vi "S4CCS.vi"() -> ()   [LabVIEW 2018]
uses:
  Channel/Channel.lvclass
  Channel/Channel.lvclass/Channel.ctl
  Header content/Header content.lvclass/Header content.ctl
  Server/Server.lvclass/Server.ctl
  Simulated_CCD_Camera/Simulated Camera.lvclass/Simulated Camera.ctl
  State Machine/CCS_State Machine.lvclass
  RxTx/CCS_RxTx.lvclass
  Simulated_CCD_Camera/Simulated Camera.lvclass
  Header content/Header content.lvclass
  Log File/CCS_Log File.lvclass
  Error log/Error log.lvclass
  Keywords Log File/Keywords Log File.lvclass
  Server/Server.lvclass
  <userlib>/gfitsio/gfitsio-read-image-subset-i32-2d.vi
panel:
  out "error out":errorcluster
  in  "Tab Control":T1(tab)
  out "S4GUI":bool
  out "S4ICS":bool
  out "TCS":bool
  out "Weather Station":bool
  out "Focuser":bool
  in  "Configuration to initialize ACS":T2={"Image path"=path "C:/images/today", "Remote IP"="200.131.64.25", "Channel"=1, "ACS mode"=0, "Communication"=0} {"Communication" items=["ZeroMQ", "TCP-IP"]; "ACS mode" items=["simulated", "real"]; "Channel" min=1 max=4}
  out "Wait expose cmd":bool
  in  "Stop Button":bool
  in  "Software version":string="v1.51.2"
  out "CCD ON/OFF":bool
  in  "use config file":bool=TRUE
  out "Acquiring 3":bool
  out "Numeric 2":i32
  out "Error Message":string
  out "Acquiring 2":bool
  out "Numeric":i32
  out "Code error message":string
  in  "clean error":bool
  out "#cycles":u32
  out "cycles done":u16
  out "#seqs":u32
  out "seqs done":u16
  out "last update":string
  out "S4GUI Message":string
  out "Last image":string
  out "frames done":u16
  out "CCD status":string
  out "Temperature (ºC)":i16
  out "Temperature status":string
  out "exptime (s)":dbl
  out "Serial number":u16
  out "Acquiring":bool
  out "#frames":u32
  in  "video mode":bool
  in  "reset axis":bool
  in  "contrast":dbl(slide)=1.0 scale=0.0..1.0
  in  "counts level":dbl(slide)=15.0 scale=0.0..5.0
  out "Intensity Graph":u16[][](graph)
  out "Header CCD Config":T3={"EM_GAIN"=2, "FRAME_TRANSFER"=TRUE, "SHUTTER_OPENING_TIME"=50, "SHUTTER_CLOSING_TIME"=50, "VBIN"=1, "INITIAL_LINE"=1, "INITIAL_COLUMN"=1, "FINAL_LINE"=1024, "FINAL_COLUMN"=1024, "HBIN"=1, "AD_CHANNEL"=0, "EM_MODE"=1, "PREAMP"=0, "SHUTTER_TTL"=0, "SHUTTER_MODE"=2, "ACQUISITION_MODE"=3, "TRIGGER_MODE"=0, "VERTICAL_CLOCK_VOLTAGE"=0, "VERTICAL_SHIFT_SPEED"=3, "READ_MODE"=4, "Last update"=timestamp(0 s since 1904-01-01), "READOUT_RATE"=""} {"READ_MODE" items=["Full Vertical Binning", "Multi-track", "Random-track", "Single-track", "Image"]; "VERTICAL_SHIFT_SPEED" items=["0.6", "1.13", "2.2", "4.33"]; "VERTICAL_CLOCK_VOLTAGE" items=["0", "+1", "+2", "+3", "+4"]; "TRIGGER_MODE" items=["Internal", "External", "N/A", "N/A_1", "N/A_2", "N/A_3", "External Start"]; "ACQUISITION_MODE" items=["Reserved", "Single", "Accumulate", "Kinetic"]; "SHUTTER_MODE" items=["Auto", "Open", "Closed"]; "SHUTTER_TTL" items=["TTL Low", "TTL High"]; "PREAMP" items=["Gain 1", "Gain 2"]; "EM_MODE" items=["Electron Multiplying", "Conventional"]}
  out "ACS status":string
  out "S4GUI":string
  out "S4ICS":string
  out "TCS":string
  out "Focuser":string
  out "Weather station":string
  in  "Channel.lvclass":refnum<class "Channel.lvclass">
  # "SPARC4 Camera Control System (S4CCS)"
  # "Init communication"
  # "CCD status"
  # "Security error:"
  # "Execution error:"
  # "x1000"
  # "Camera configuration"
  # "Communication with the sub-systems of the observatory"
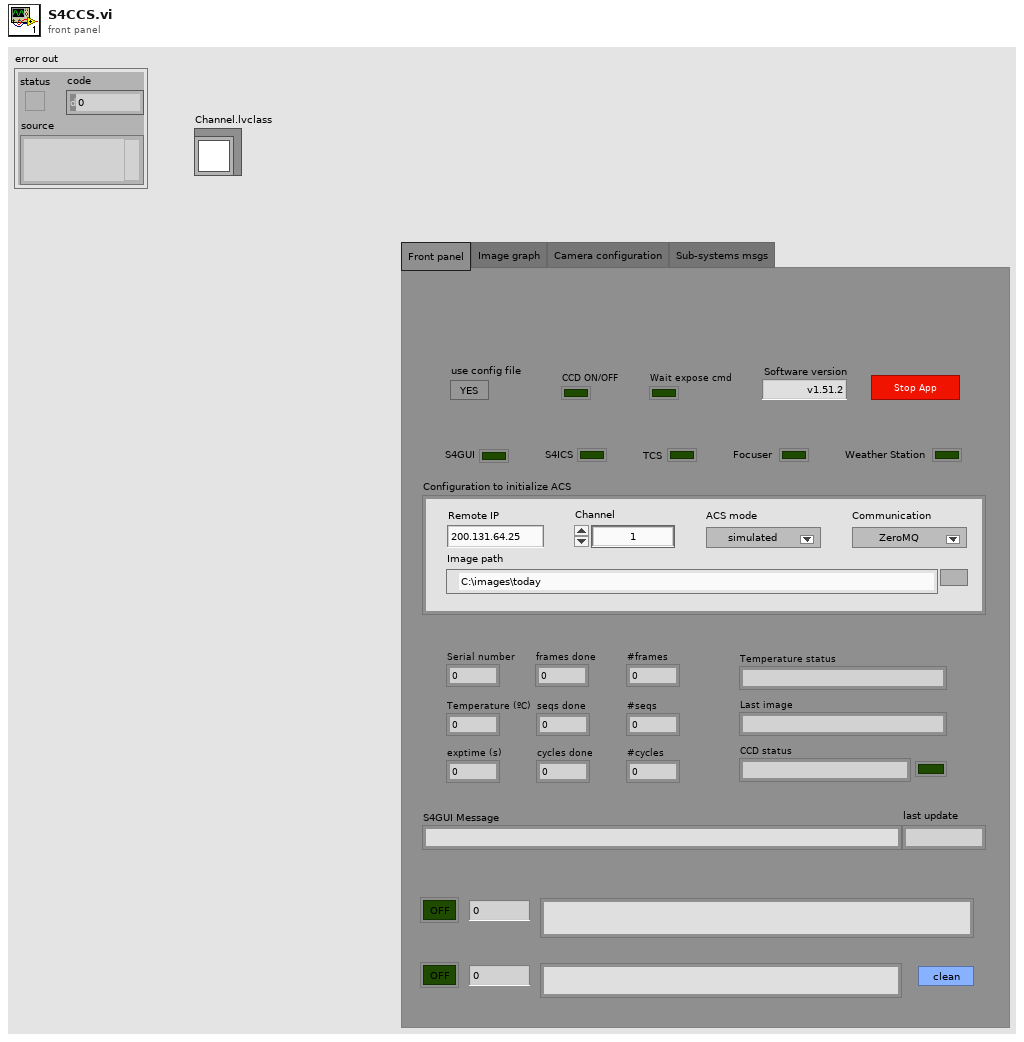
[diagram p1: front panel]
types:
  T1 = enum32{"Front panel", "Image graph", "Camera configuration", "Sub-systems msgs"}
  T2 = cluster{"Image path":path, "Remote IP":string, "Channel":u8, "ACS mode":u16, "Communication":u16}
  T3 = cluster{"EM_GAIN":u16, "FRAME_TRANSFER":bool, "SHUTTER_OPENING_TIME":u16, "SHUTTER_CLOSING_TIME":u16, "VBIN":u16, "INITIAL_LINE":u16, "INITIAL_COLUMN":u16, "FINAL_LINE":u16, "FINAL_COLUMN":u16, "HBIN":u16, "AD_CHANNEL":u16, "EM_MODE":u16, "PREAMP":u16, "SHUTTER_TTL":u16, "SHUTTER_MODE":u16, "ACQUISITION_MODE":u16, "TRIGGER_MODE":u16, "VERTICAL_CLOCK_VOLTAGE":u16, "VERTICAL_SHIFT_SPEED":u16, "READ_MODE":u16, "Last update":timestamp, "READOUT_RATE":string}
  T4 = cluster{"Stop Acquisition":bool, "Abort Acquisition":bool, "Pause acquisition":bool, "wait expose command":bool, "video mode":bool}
  T5 = cluster{"State Machine.lvclass":refnum<class "CCS_State Machine.lvclass">, "RxTx.lvclass":refnum<class "CCS_RxTx.lvclass">, "Simulated_CCD_Camera.lvclass":refnum<class "Simulated Camera.lvclass">, "Save_Header_RxTx.lvclass":refnum<class "CCS_RxTx.lvclass">, "Header Content.lvclass":refnum<class "Header content.lvclass">, "Status SM.lvclass":refnum<class "CCS_State Machine.lvclass">, "Status RxTx.lvclass":refnum<class "CCS_RxTx.lvclass">, "Log File.lvclass":refnum<class "CCS_Log File.lvclass">, "Error log.lvclass":refnum<class "Error log.lvclass">, "Keywords Log File.lvclass":refnum<class "Keywords Log File.lvclass">}
  T6 = cluster{"CYCLES_DONE":u16, "LAST_IMAGE_NAME":string, "DISK_SPACE":u16, "FRAMES_DONE":u16, "CCD_STATUS":string, "CURRENT_TEMPERATURE":i16, "TEMPERATURE_STATUS":string, "FRAME_EXPOSURE_TIME":sgl, "ERROR":bool, "SERIAL_NUMBER":u16, "ACQUIRING":bool, "IMAGE_INDEX":u32, "SEQS_DONE":u16}
  T7 = cluster{"COOLER_POWER_STATUS":u16, "TEMP":i32, "EXPTIME":dbl, "#FRAMES":u32, "#CYCLES":u32, "#SEQS":u32, "WAVEPLATE_POS":u16}
  T8 = cluster{"PREAMP":u16, "READOUT_RATE":u16, "EM_GAIN":u16, "VERTICAL_SHIFT_SPEED":u16, "READ_MODE":u16, "FRAME_TRANSFER":bool, "VERTICAL_CLOCK_VOLTAGE":u16, "ACQUISITION_MODE":u16, "AD_CHANNEL":u16, "EM_MODE":u16, "SHUTTER_TTL":u16, "SHUTTER_OPENING_TIME":u16, "SHUTTER_CLOSING_TIME":u16, "SHUTTER_MODE":u16, "TRIGGER_MODE":u16, "VBIN":u16, "INITIAL_LINE":u16, "INITIAL_COLUMN":u16, "FINAL_LINE":u16, "FINAL_COLUMN":u16, "HBIN":u16}
  T9 = cluster{"CCD status":string, "CCD configuration":string, "Acquisition configuration":string, "S4GUI JSON string":string}
  T10 = typedef "gfitsio.lvlib/gfitsio-refnum.ctl" = refnum<k1>
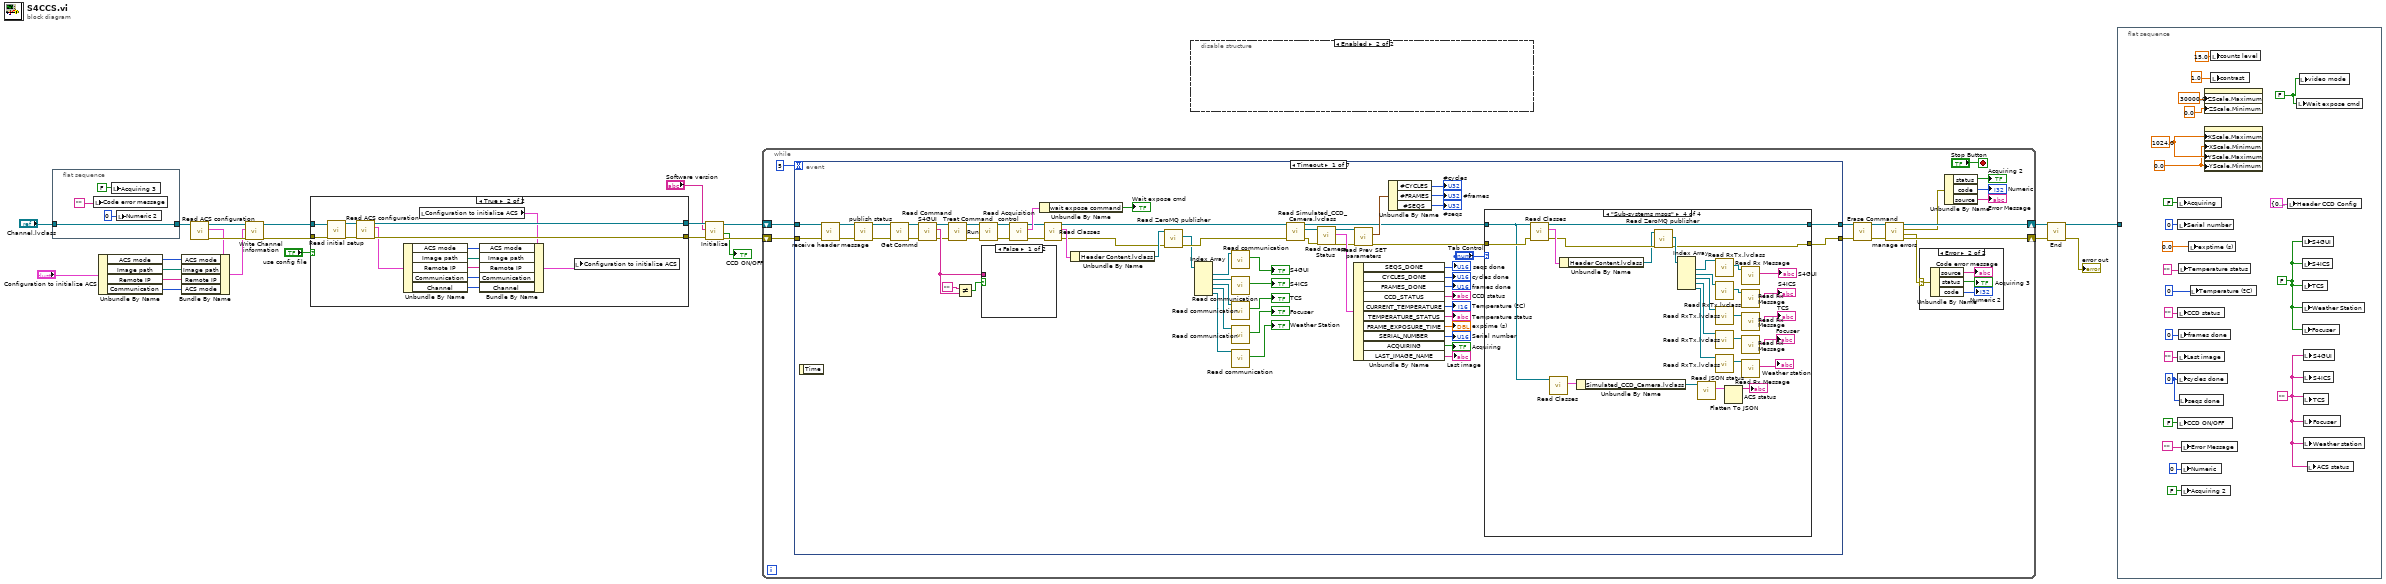
[diagram p0: block diagram]
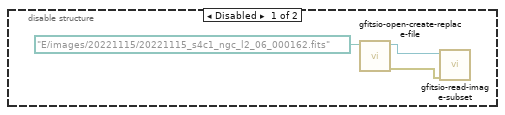
[diagram p3: hidden frame]
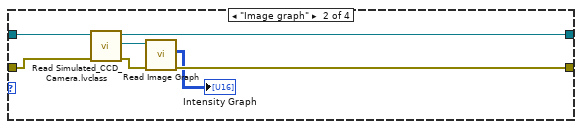
[diagram p6: hidden frame]
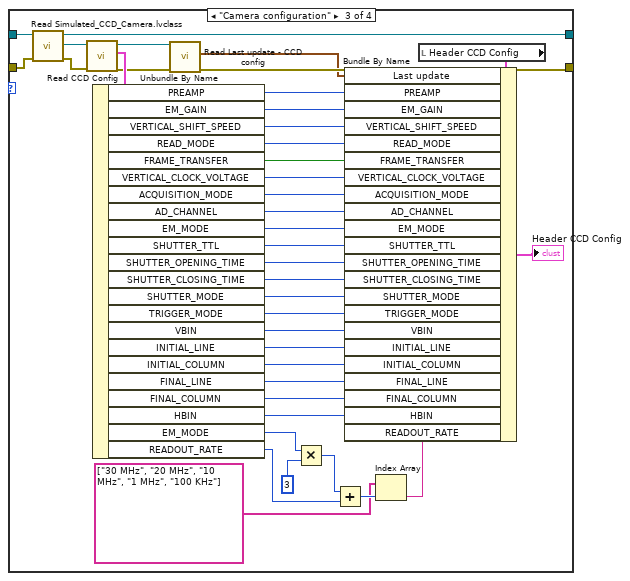
[diagram p7: hidden frame]
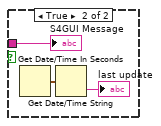
[diagram p8: hidden frame]
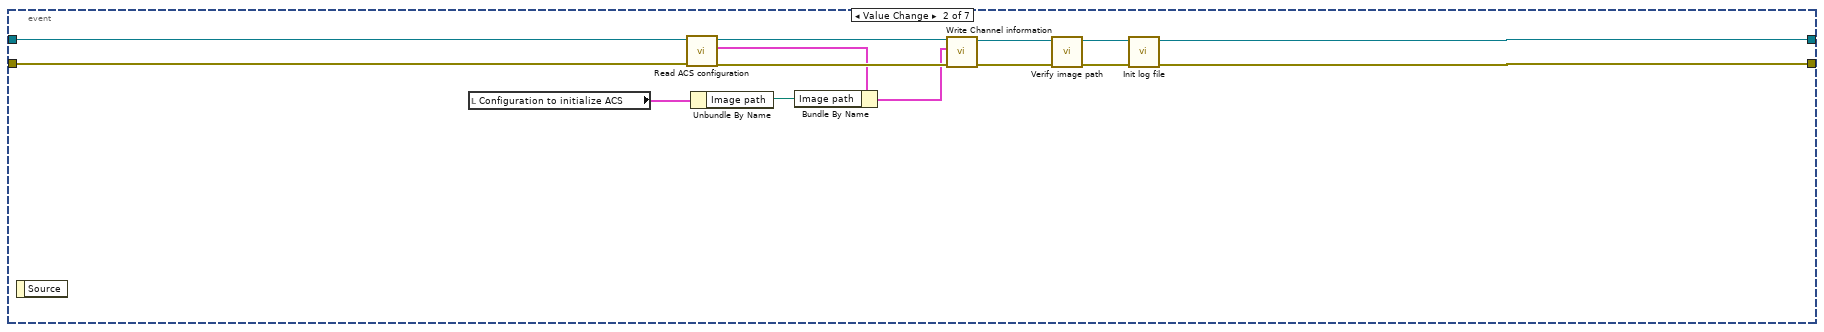
[diagram p9: hidden frame]
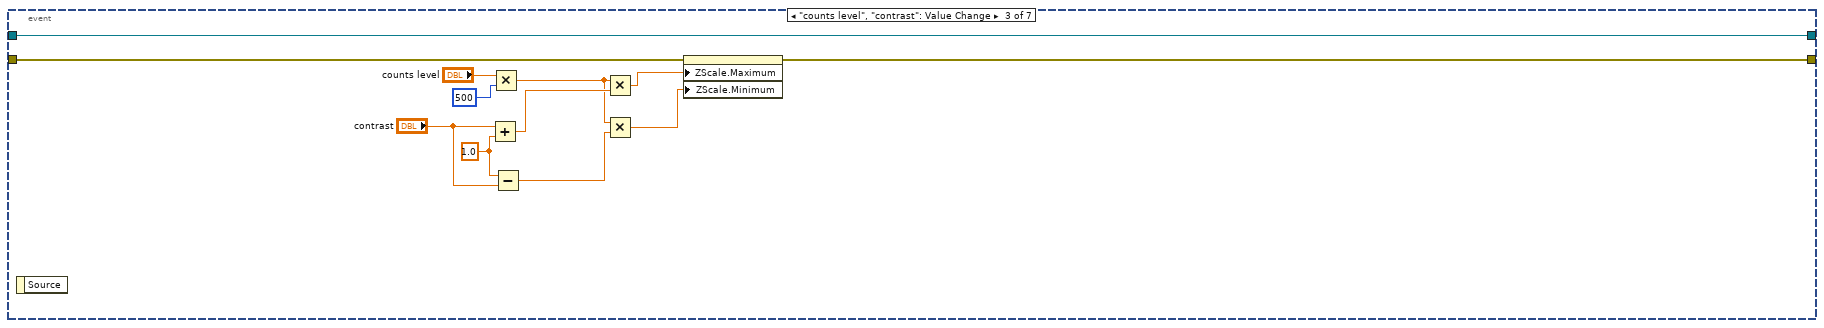
[diagram p10: hidden frame]
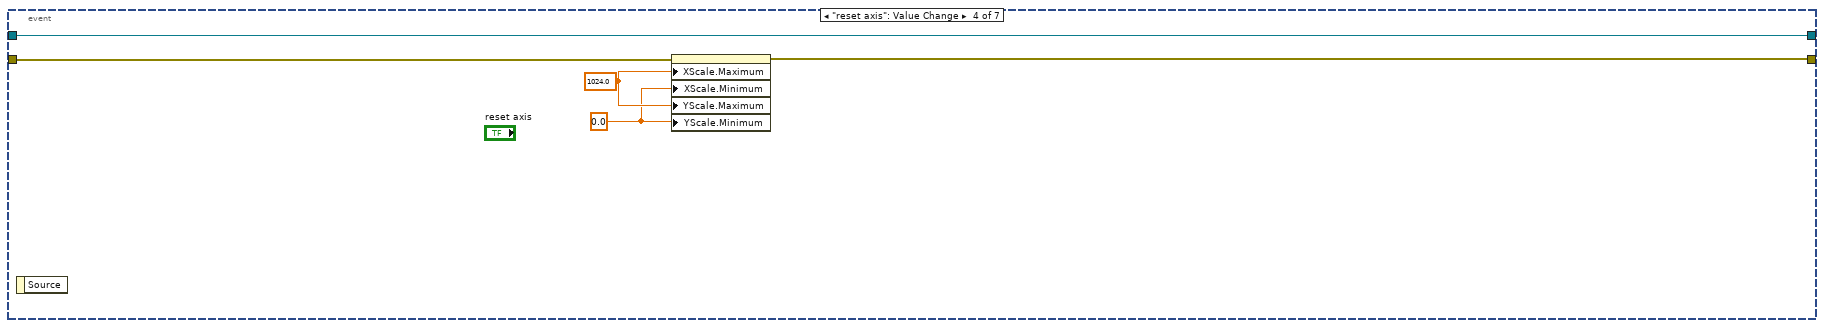
[diagram p11: hidden frame]
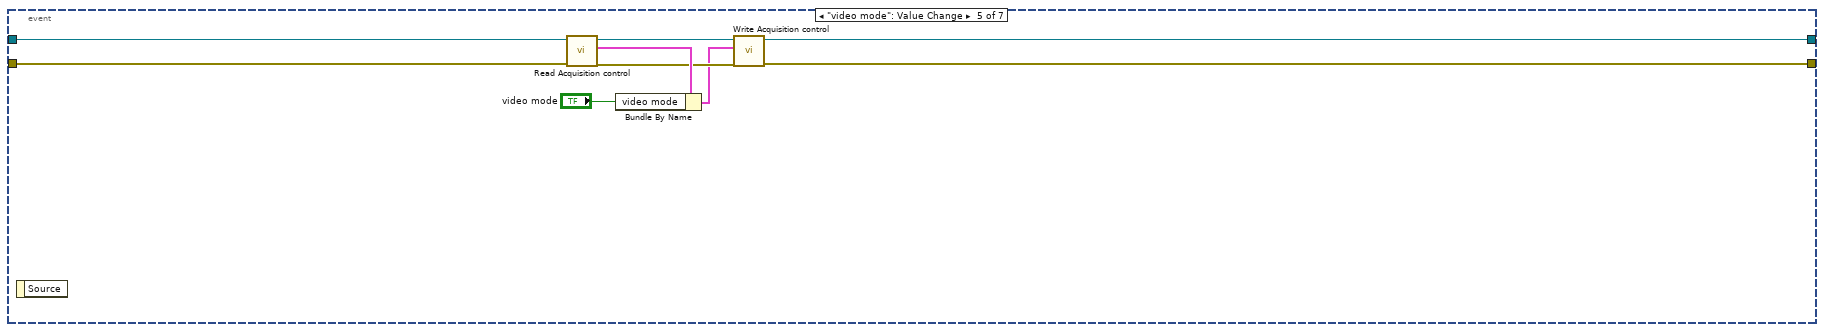
[diagram p12: hidden frame]
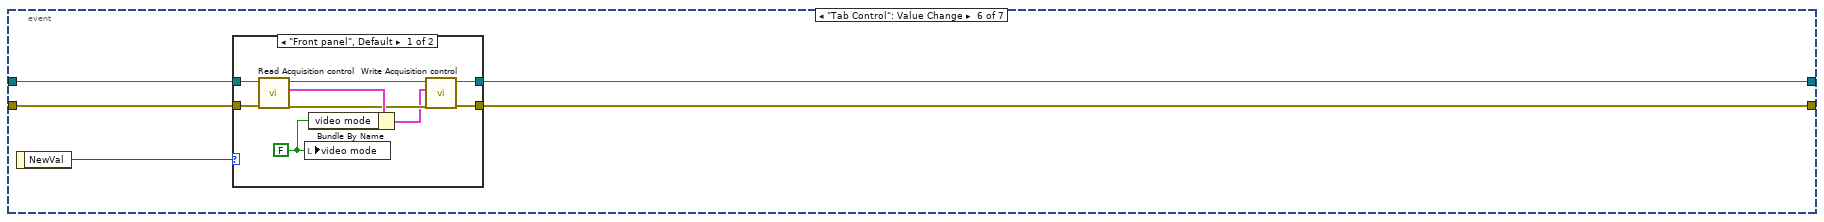
[diagram p13: hidden frame]
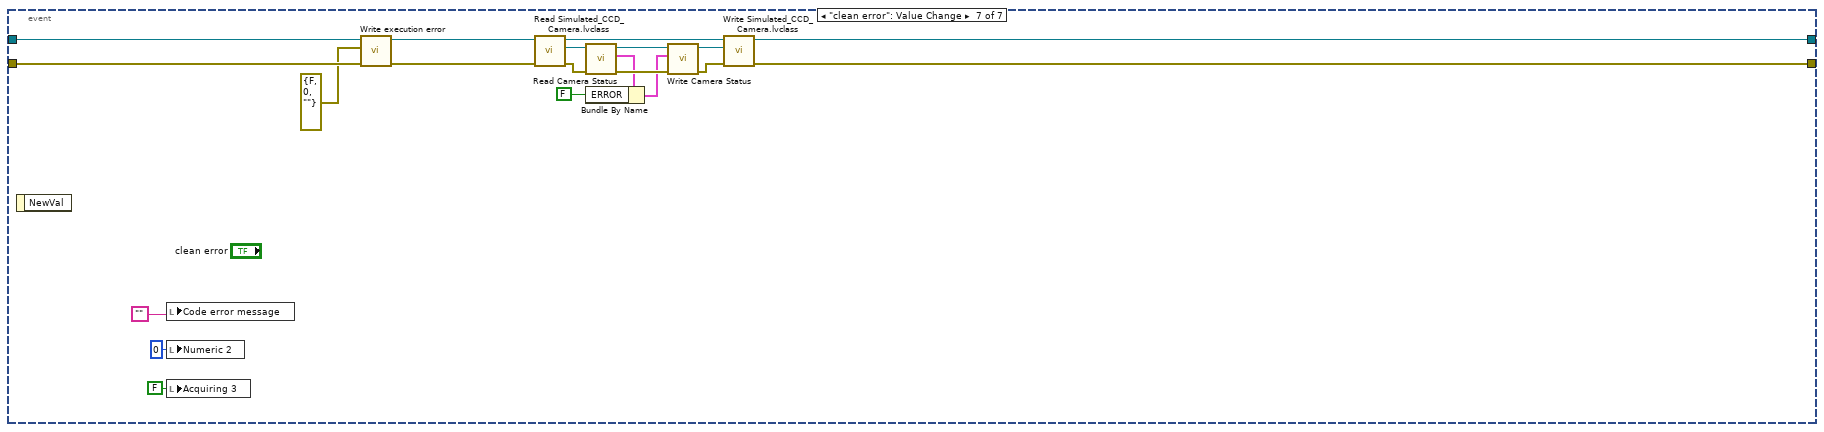
[diagram p15: hidden frame]
diagram:
  n1 = flat-sequence {
    tunnel: "Channel.lvclass" -> [w28]
    tunnel: [w28] -> w11
    frame #0 {
      n2 = local write "Code error message"("") -> ()
      n3 = local write "Acquiring 3"(FALSE ("Acquiring 3")) -> ()
      n4 = local write "Numeric 2"(0 ("Numeric 2")) -> ()
    }
  }
  n5 = Unbundle By Name("Configuration to initialize ACS") -> ("ACS mode"=w5:u16, "Image path"=w4:path, "Remote IP"=w3:string, "Communication"=w2:u16)
  n6 = call-dynamic "Read ACS configuration.vi"("Channel in"=w11) -> ("error out"=w9:errorcluster, "acs init configuration"=w8:T2, "Channel out"=w10:refnum<class "Channel.lvclass">)  [unwired: 8 in]
  n7 = Bundle By Name(cluster=w8, "ACS mode"=w5, "Image path"=w4, "Remote IP"=w3, "ACS mode"=w2) -> (w7:T2)
  n8 = call-dynamic "Write Channel information.vi"("error in (no error)"=w9, "acs init configuration"=w7, "Channel in"=w10) -> ("error out"=w15:errorcluster, "Channel out"=w16:refnum<class "Channel.lvclass">)  [unwired: 7 in]
  n9 = case shown="True" "use config file" {
    tunnel: w16 -> [w30 w44]
    tunnel: w15 -> [w29 w43]
    tunnel: [w30 w40] -> w14
    tunnel: [w29 w39] -> w13
    frame False {
    }
    frame True {
      n10 = call "Read initial setup.vi"("error in (no error)"=w43, "Channel in"=w44) -> ("error out"=w41:errorcluster, "Channel out"=w42:refnum<class "Channel.lvclass">)  [unwired: 8 in]
      n11 = call-dynamic "Read ACS configuration.vi"("error in (no error)"=w41, "Channel in"=w42) -> ("error out"=w39:errorcluster, "acs init configuration"=w38:T2, "Channel out"=w40:refnum<class "Channel.lvclass">)  [unwired: 7 in]
      n12 = Unbundle By Name(w38) -> ("ACS mode"=w32:u16, "Image path"=w33:path, "Remote IP"=w34:string, "Communication"=w35:u16, "Channel"=w31:u8)
      n13 = local read "Configuration to initialize ACS"() -> (w36:T2)
      n14 = Bundle By Name(cluster=w36, "ACS mode"=w32, "Image path"=w33, "Remote IP"=w34, "Communication"=w35, "Channel"=w31) -> (w37:T2)
      n15 = local write "Configuration to initialize ACS"(w37) -> ()
    }
  }
  n16 = call "Initialize.vi"("error IO"=w13, "Software version"="Software version", "Channel.lvclass"=w14) -> ("error IO 2"=w24:errorcluster, "Initialization"=→"CCD ON/OFF":bool, "Channel.lvclass 2"=w23:refnum<class "Channel.lvclass">)  [unwired: 6 in]
  n17 = while {
    shift-right: [w52] -> w21
    shift-left: w24 -> [w58]
    shift-right: [w54] -> w22
    shift-left: w23 -> [w59]
    stop <- "Stop Button" stop-if-true
    n18 = event shown="[0] Timeout" {
      selector: _ -> [_ _ _ _ _ _ _]
      dyn-events: _ -> [_ _ _ _ _ _ _]
      timeout: 5 -> [_ _ _ _ _ _ _]
      tunnel: [w100 w203 w226 w231 w236 w244 w259] -> w46
      tunnel: [w64 w204 w228 w233 w237 w243 w260] -> w47
      tunnel: w59 -> [w95 w215 w228 w233 w239 w246 w274]
      tunnel: w58 -> [w94 w214 w227 w232 w238 w245 w275]
      event Timeout {
        n19 = event-data() -> ()  [unwired: 1 in, 1 out]
        n20 = call "receive header message.vi"("error in (no error)"=w94, "Channel in"=w95) -> ("error out"=w93:errorcluster, "Channel out"=w92:refnum<class "Channel.lvclass">)  [unwired: 8 in]
        n21 = call "publish status.vi"("error in (no error)"=w93, "Channel in"=w92) -> ("error out"=w96:errorcluster, "Channel out"=w97:refnum<class "Channel.lvclass">)  [unwired: 8 in]
        n22 = call "Get Commd.vi"("error in (no error)"=w96, "Channel in"=w97) -> ("error out"=w109:errorcluster, "Channel out"=w110:refnum<class "Channel.lvclass">)  [unwired: 8 in]
        n23 = call "Read Command S4GUI.vi"("error in (no error)"=w109, "Channel in"=w110) -> ("error out"=w84:errorcluster, "Message"=w123:string, "Channel out"=w85:refnum<class "Channel.lvclass">)  [unwired: 7 in]
        n24 = call "Treat Command.vi"("error in (no error)"=w84, "Channel in"=w85) -> ("error out"=w87:errorcluster, "Channel out"=w86:refnum<class "Channel.lvclass">)  [unwired: 8 in]
        n25 = Not Equal?(x="", y=w123) -> (x != y?=w124:bool)
        n26 = call "Run.vi"("error in (no error)"=w87, "Channel in"=w86) -> ("error out"=w121:errorcluster, "Channel out"=w120:refnum<class "Channel.lvclass">)  [unwired: 8 in]
        n27 = case shown="False" w124 {
          tunnel: w123 -> [_ w202]
          frame False {
          }
          frame True {
            n28 = Get Date/Time In Seconds() -> (seconds since 1Jan1904=w201:timestamp)
            n29 = Get Date/Time String(seconds (now)=w201) -> (time string=→"last update":string)  [unwired: 2 in, 1 out]
            "S4GUI Message" <- w202
          }
        }
        n30 = call "Read Acquisition control.vi"("error in (no error)"=w121, "Channel in"=w120) -> ("error out"=w83:errorcluster, "Acquisition control"=w91:T4, "Channel out"=w82:refnum<class "Channel.lvclass">)  [unwired: 7 in]
        n31 = Unbundle By Name(w91) -> ("wait expose command"=→"Wait expose cmd":bool)
        n32 = call "Read Classes.vi"("error in (no error)"=w83, "Channel in"=w82) -> ("error out"=w79:errorcluster, "Classes"=w81:T5, "Channel out"=w78:refnum<class "Channel.lvclass">)  [unwired: 7 in]
        n33 = Unbundle By Name(w81) -> ("Header Content.lvclass"=w80:refnum<class "Header content.lvclass">)
        n34 = call "Read ZeroMQ publisher.vi"("error in (no error)"=w79, "Header content in"=w80) -> ("error out"=w77:errorcluster, "ZeroMQ publisher"=w76:refnum<class "Server.lvclass">[])  [unwired: 7 in, 1 out]
        n35 = Index Array(array=w76) -> (element #1=w75:refnum<class "Server.lvclass">, element #2=w74:refnum<class "Server.lvclass">, element #3=w73:refnum<class "Server.lvclass">, element #4=w72:refnum<class "Server.lvclass">, element #5=w71:refnum<class "Server.lvclass">)  [unwired: 5 in]
        n36 = call "Read communication.vi"("Server in"=w71) -> ("communication"=→"Weather Station":bool)  [unwired: 8 in, 2 out]
        n37 = call "Read communication.vi"("Server in"=w75) -> ("communication"=→"S4GUI":bool)  [unwired: 8 in, 2 out]
        n38 = call "Read communication.vi"("Server in"=w74) -> ("communication"=→"S4ICS":bool)  [unwired: 8 in, 2 out]
        n39 = call "Read communication.vi"("Server in"=w73) -> ("communication"=→"TCS":bool)  [unwired: 8 in, 2 out]
        n40 = call "Read communication.vi"("Server in"=w72) -> ("communication"=→"Focuser":bool)  [unwired: 8 in, 2 out]
        n41 = call "Read Simulated_CCD_Camera.lvclass.vi"("error in (no error)"=w77, "Channel in"=w78) -> ("error out"=w89:errorcluster, "Simulated_CCD_Camera.lvclass"=w88:refnum<class "Simulated Camera.lvclass">, "Channel out"=w65:refnum<class "Channel.lvclass">)  [unwired: 7 in]
        n42 = call "Read Camera Status.vi"("error in (no error)"=w89, "CCDCamera in"=w88) -> ("error out"=w105:errorcluster, "Camera Status"=w119:T6, "CCDCamera out"=w106:refnum<class "Simulated Camera.lvclass">)  [unwired: 7 in]
        n43 = Unbundle By Name(w119) -> ("SEQS_DONE"=→"seqs done":u16, "CYCLES_DONE"=→"cycles done":u16, "FRAMES_DONE"=→"frames done":u16, "CCD_STATUS"=→"CCD status":string, "CURRENT_TEMPERATURE"=→"Temperature (ºC)":i16, "TEMPERATURE_STATUS"=→"Temperature status":string, "FRAME_EXPOSURE_TIME"=→"exptime (s)":sgl, "SERIAL_NUMBER"=→"Serial number":u16, "ACQUIRING"=→"Acquiring":bool, "LAST_IMAGE_NAME"=→"Last image":string)
        n44 = call-dynamic "Read Prev SET parameters.vi"("error in (no error)"=w105, "Simulated_CCD_Camera in"=w106) -> ("error out"=w101:errorcluster, "Prev SET parameters"=w104:T7)  [unwired: 7 in, 1 out]
        n45 = Unbundle By Name(w104) -> ("#CYCLES"=→"#cycles":u32, "#FRAMES"=→"#frames":u32, "#SEQS"=→"#seqs":u32)
        n46 = case shown="\"Sub-systems msgs\"" "Tab Control" {
          tunnel: w101 -> [w126 w130 w137 w199]
          tunnel: [w126 w133 w147 w193] -> w100
          tunnel: w65 -> [w125 w131 w138 w177]
          tunnel: [w125 w127 w134 w196] -> w64
          frame "Front panel", Default {
          }
          frame "Image graph" {
            n47 = call "Read Simulated_CCD_Camera.lvclass.vi"("error in (no error)"=w130, "Channel in"=w131) -> ("error out"=w129:errorcluster, "Simulated_CCD_Camera.lvclass"=w128:refnum<class "Simulated Camera.lvclass">, "Channel out"=w127:refnum<class "Channel.lvclass">)  [unwired: 7 in]
            n48 = call "Read Image Graph.vi"("error in (no error)"=w129, "CCDCamera in"=w128) -> ("error out"=w133:errorcluster, "Image Graph"=→"Intensity Graph":u16[][])  [unwired: 7 in, 1 out]
          }
          frame "Camera configuration" {
            n49 = call "Read Simulated_CCD_Camera.lvclass.vi"("error in (no error)"=w137, "Channel in"=w138) -> ("error out"=w136:errorcluster, "Simulated_CCD_Camera.lvclass"=w135:refnum<class "Simulated Camera.lvclass">, "Channel out"=w134:refnum<class "Channel.lvclass">)  [unwired: 7 in]
            n50 = call "Read CCD Config.vi"("error in (no error)"=w136, "CCDCamera in"=w135) -> ("error out"=w148:errorcluster, "CCD Config"=w172:T8, "CCDCamera out"=w149:refnum<class "Simulated Camera.lvclass">)  [unwired: 7 in]
            n51 = Unbundle By Name(w172) -> ("PREAMP"=w171:u16, "EM_GAIN"=w170:u16, "VERTICAL_SHIFT_SPEED"=w157:u16, "READ_MODE"=w156:u16, "FRAME_TRANSFER"=w169:bool, "VERTICAL_CLOCK_VOLTAGE"=w155:u16, "ACQUISITION_MODE"=w154:u16, "AD_CHANNEL"=w168:u16, "EM_MODE"=w153:u16, "SHUTTER_TTL"=w152:u16, "SHUTTER_OPENING_TIME"=w167:u16, "SHUTTER_CLOSING_TIME"=w166:u16, "SHUTTER_MODE"=w151:u16, "TRIGGER_MODE"=w150:u16, "VBIN"=w165:u16, "INITIAL_LINE"=w164:u16, "INITIAL_COLUMN"=w163:u16, "FINAL_LINE"=w162:u16, "FINAL_COLUMN"=w161:u16, "HBIN"=w160:u16, "EM_MODE"=w145:u16, "READOUT_RATE"=w142:u16)
            n52 = call-dynamic "Read Last update - CCD config.vi"("error in (no error)"=w148, "Simulated_CCD_Camera in"=w149) -> ("error out"=w147:errorcluster, "Last update - CCD config"=w146:timestamp)  [unwired: 7 in, 1 out]
            n53 = Multiply(x=w145, y=3) -> (x*y=w143:i32)
            n54 = Add(x=w143, y=w142) -> (x+y=w141:i32)
            n55 = Index Array(array=string[] ["30 MHz", "20 MHz", "10 MHz", "1 MHz", "100 KHz"], index=w141) -> (element=w140:string)
            n56 = local read "Header CCD Config"() -> (w158:T3)
            n57 = Bundle By Name(cluster=w158, "Last update"=w146, "PREAMP"=w171, "EM_GAIN"=w170, "VERTICAL_SHIFT_SPEED"=w157, "READ_MODE"=w156, "FRAME_TRANSFER"=w169, "VERTICAL_CLOCK_VOLTAGE"=w155, "ACQUISITION_MODE"=w154, "AD_CHANNEL"=w168, "EM_MODE"=w153, "SHUTTER_TTL"=w152, "SHUTTER_OPENING_TIME"=w167, "SHUTTER_CLOSING_TIME"=w166, "SHUTTER_MODE"=w151, "TRIGGER_MODE"=w150, "VBIN"=w165, "INITIAL_LINE"=w164, "INITIAL_COLUMN"=w163, "FINAL_LINE"=w162, "FINAL_COLUMN"=w161, "HBIN"=w160, "READOUT_RATE"=w140) -> (→"Header CCD Config":T3)
          }
          frame "Sub-systems msgs" {
            n58 = call "Read Classes.vi"("error in (no error)"=w199, "Channel in"=w177) -> ("error out"=w197:errorcluster, "Classes"=w198:T5, "Channel out"=w196:refnum<class "Channel.lvclass">)  [unwired: 7 in]
            n59 = call "Read Classes.vi"("Channel in"=w177) -> ("Classes"=w176:T5)  [unwired: 8 in, 2 out]
            n60 = Unbundle By Name(w198) -> ("Header Content.lvclass"=w195:refnum<class "Header content.lvclass">)
            n61 = Unbundle By Name(w176) -> ("Simulated_CCD_Camera.lvclass"=w175:refnum<class "Simulated Camera.lvclass">)
            n62 = call "Read ZeroMQ publisher.vi"("error in (no error)"=w197, "Header content in"=w195) -> ("error out"=w193:errorcluster, "ZeroMQ publisher"=w194:refnum<class "Server.lvclass">[])  [unwired: 7 in, 1 out]
            n63 = Index Array(array=w194) -> (element #1=w192:refnum<class "Server.lvclass">, element #2=w191:refnum<class "Server.lvclass">, element #3=w190:refnum<class "Server.lvclass">, element #4=w189:refnum<class "Server.lvclass">, element #5=w188:refnum<class "Server.lvclass">)  [unwired: 5 in]
            n64 = call "Read JSON status.vi"("Simulated_CCD_Camera in"=w175) -> ("JSON status"=w173:T9)  [unwired: 8 in, 2 out]
            n65 = call "Read RxTx.lvclass.vi"("Server in"=w192) -> ("RxTx.lvclass"=w187:refnum<class "CCS_RxTx.lvclass">)  [unwired: 8 in, 2 out]
            n66 = call "Read RxTx.lvclass.vi"("Server in"=w191) -> ("RxTx.lvclass"=w186:refnum<class "CCS_RxTx.lvclass">)  [unwired: 8 in, 2 out]
            n67 = call "Read RxTx.lvclass.vi"("Server in"=w190) -> ("RxTx.lvclass"=w185:refnum<class "CCS_RxTx.lvclass">)  [unwired: 8 in, 2 out]
            n68 = call "Read RxTx.lvclass.vi"("Server in"=w189) -> ("RxTx.lvclass"=w184:refnum<class "CCS_RxTx.lvclass">)  [unwired: 8 in, 2 out]
            n69 = call "Read RxTx.lvclass.vi"("Server in"=w188) -> ("RxTx.lvclass"=w183:refnum<class "CCS_RxTx.lvclass">)  [unwired: 8 in, 2 out]
            n70 = Flatten To JSON(anything=w173) -> (JSON string=→"ACS status":string)  [unwired: 2 in, 1 out]
            n71 = call "Read Rx Message.vi"("RxTx in"=w187) -> ("Rx Message"=→"S4GUI":string)  [unwired: 8 in, 2 out]
            n72 = call "Read Rx Message.vi"("RxTx in"=w186) -> ("Rx Message"=→"S4ICS":string)  [unwired: 8 in, 2 out]
            n73 = call "Read Rx Message.vi"("RxTx in"=w185) -> ("Rx Message"=→"TCS":string)  [unwired: 8 in, 2 out]
            n74 = call "Read Rx Message.vi"("RxTx in"=w184) -> ("Rx Message"=→"Focuser":string)  [unwired: 8 in, 2 out]
            n75 = call "Read Rx Message.vi"("RxTx in"=w183) -> ("Rx Message"=→"Weather station":string)  [unwired: 8 in, 2 out]
          }
        }
      }
      event "Configuration to initialize ACS.Image path": Value Change {
        n76 = event-data() -> ()  [unwired: 1 in, 1 out]
        n77 = local read "Configuration to initialize ACS"() -> (w216:T2)
        n78 = call-dynamic "Read ACS configuration.vi"("error in (no error)"=w214, "Channel in"=w215) -> ("error out"=w212:errorcluster, "acs init configuration"=w211:T2, "Channel out"=w213:refnum<class "Channel.lvclass">)  [unwired: 7 in]
        n79 = Unbundle By Name(w216) -> ("Image path"=w207:path)
        n80 = Bundle By Name(cluster=w211, "Image path"=w207) -> (w210:T2)
        n81 = call-dynamic "Write Channel information.vi"("error in (no error)"=w212, "acs init configuration"=w210, "Channel in"=w213) -> ("error out"=w208:errorcluster, "Channel out"=w209:refnum<class "Channel.lvclass">)  [unwired: 7 in]
        n82 = call "Verify image path.vi"("error in (no error)"=w208, "Channel in"=w209) -> ("error out"=w206:errorcluster, "Channel out"=w205:refnum<class "Channel.lvclass">)  [unwired: 8 in]
        n83 = call "Init log file.vi"("error in (no error)"=w206, "Channel in"=w205) -> ("error out"=w203:errorcluster, "Channel out"=w204:refnum<class "Channel.lvclass">)  [unwired: 8 in]
      }
      event "counts level", "contrast": Value Change {
        w220 = 1.0
        n84 = event-data() -> ()  [unwired: 1 in, 1 out]
        n85 = Add(x="contrast", y=w220) -> (x+y=w223:dbl)
        n86 = Multiply(x="counts level", y=500) -> (x*y=w218:dbl)
        n87 = Subtract(x=w220, y="contrast") -> (x-y=w219:dbl)
        n88 = Multiply(x=w218, y=w223) -> (x*y=w222:dbl)
        n89 = Multiply(x=w218, y=w219) -> (x*y=w221:dbl)
        n90 = property on="Intensity Graph" class="IntGraph (strict)"(error in=w227, "ZScale.Maximum"=w222, "ZScale.Minimum"=w221) -> (error out=w226:errorcluster)  [unwired: 1 in, 1 out]
      }
      event "reset axis": Value Change {
        w229 = 0.0
        w230 = 1024.0
        n91 = event-data() -> ()  [unwired: 1 in, 1 out]
        n92 = property on="Intensity Graph" class="IntGraph (strict)"(error in=w232, "XScale.Maximum"=w230, "XScale.Minimum"=w229, "YScale.Maximum"=w230, "YScale.Minimum"=w229) -> (error out=w231:errorcluster)  [unwired: 1 in, 1 out]
      }
      event "video mode": Value Change {
        n93 = event-data() -> ()  [unwired: 1 in, 1 out]
        n94 = call "Read Acquisition control.vi"("error in (no error)"=w238, "Channel in"=w239) -> ("error out"=w241:errorcluster, "Acquisition control"=w242:T4, "Channel out"=w240:refnum<class "Channel.lvclass">)  [unwired: 7 in]
        n95 = Bundle By Name(cluster=w242, "video mode"="video mode") -> (w235:T4)
        n96 = call "Write Acquisition control.vi"("error in (no error)"=w241, "Acquisition control"=w235, "Channel in"=w240) -> ("error out"=w236:errorcluster, "Channel out"=w237:refnum<class "Channel.lvclass">)  [unwired: 7 in]
      }
      event "Tab Control": Value Change {
        n97 = event-data() -> ("NewVal"=w247:T1)  [unwired: 1 in]
        n98 = case shown="\"Front panel\", Default" w247 {
          tunnel: w246 -> [w255 w258]
          tunnel: w245 -> [w256 w257]
          tunnel: [w254 w257] -> w244
          tunnel: [w253 w258] -> w243
          frame "Front panel", Default {
            w251 = FALSE ("video mode")
            n99 = call "Read Acquisition control.vi"("error in (no error)"=w256, "Channel in"=w255) -> ("error out"=w250:errorcluster, "Acquisition control"=w252:T4, "Channel out"=w249:refnum<class "Channel.lvclass">)  [unwired: 7 in]
            n100 = local write "video mode"(w251) -> ()
            n101 = Bundle By Name(cluster=w252, "video mode"=w251) -> (w248:T4)
            n102 = call "Write Acquisition control.vi"("error in (no error)"=w250, "Acquisition control"=w248, "Channel in"=w249) -> ("error out"=w254:errorcluster, "Channel out"=w253:refnum<class "Channel.lvclass">)  [unwired: 7 in]
          }
          frame "Image graph" {
          }
        }
      }
      event "clean error": Value Change {
        n103 = event-data() -> ()  [unwired: 1 in, 1 out]
        n104 = local write "Code error message"("") -> ()
        n105 = local write "Numeric 2"(0 ("Numeric 2")) -> ()
        n106 = local write "Acquiring 3"(FALSE ("Acquiring 3")) -> ()
        n107 = call-dynamic "Write execution error.vi"("error in (no error)"=w275, "execution error"=errorcluster {"status"=FALSE, "code"=0, "source"=""}, "Channel in"=w274) -> ("error out"=w267:errorcluster, "Channel out"=w268:refnum<class "Channel.lvclass">)  [unwired: 7 in]
        n108 = call "Read Simulated_CCD_Camera.lvclass.vi"("error in (no error)"=w267, "Channel in"=w268) -> ("error out"=w265:errorcluster, "Simulated_CCD_Camera.lvclass"=w266:refnum<class "Simulated Camera.lvclass">, "Channel out"=w261:refnum<class "Channel.lvclass">)  [unwired: 7 in]
        n109 = call "Read Camera Status.vi"("error in (no error)"=w265, "CCDCamera in"=w266) -> ("error out"=w272:errorcluster, "Camera Status"=w271:T6, "CCDCamera out"=w262:refnum<class "Simulated Camera.lvclass">)  [unwired: 7 in]
        n110 = Bundle By Name(cluster=w271, "ERROR"=FALSE) -> (w270:T6)
        n111 = call "Write Camera Status.vi"("error in (no error)"=w272, "Camera Status"=w270, "CCDCamera in"=w262) -> ("error out"=w264:errorcluster, "CCDCamera out"=w263:refnum<class "Simulated Camera.lvclass">)  [unwired: 7 in]
        n112 = call "Write Simulated_CCD_Camera.lvclass.vi"("error in (no error)"=w264, "Simulated_CCD_Camera.lvclass"=w263, "Channel in"=w261) -> ("error out"=w259:errorcluster, "Channel out"=w260:refnum<class "Channel.lvclass">)  [unwired: 7 in]
      }
    }
    n113 = call "Erase Command.vi"("error in (no error)"=w46, "Channel in"=w47) -> ("error out"=w48:errorcluster, "Channel out"=w55:refnum<class "Channel.lvclass">)  [unwired: 8 in]
    n114 = call "manage errors.vi"("error in (no error)"=w48, "Channel in"=w55) -> ("error out"=w52:errorcluster, "sys error"=w45:errorcluster, "exe error"=w53:errorcluster, "Channel out"=w54:refnum<class "Channel.lvclass">)  [unwired: 6 in]
    n115 = case shown="Error" w45 {
      selector: w45 -> [_ w60]
      frame No Error {
      }
      frame Error {
        n116 = Unbundle By Name(w60) -> ("source"=→"Code error message":string, "status"=→"Acquiring 3":bool, "code"=→"Numeric 2":i32)
      }
    }
    n117 = Unbundle By Name(w53) -> ("status"=→"Acquiring 2":bool, "code"=→"Numeric":i32, "source"=→"Error Message":string)
  }
  n118 = disable-structure shown="Enabled" {
    frame Disabled {
      n119 = call <userlib>:"gfitsio-open-create-replace-file.vi"("file path (dialog if empty)"=path "E:/images/20221115/20221115_s4c1_ngc_l2_06_000162.fits") -> ("error out"=w280:errorcluster, "gfits refnum"=w281:T10)  [unwired: 8 in, 1 out]
      n120 = call-poly <userlib>:"gfitsio-read-image-subset.vi"("error in (no error)"=w280, "gfits refnum"=w281) -> ()  [unwired: 7 in, 3 out]
    }
    frame Enabled {
    }
  }
  n121 = call "End.vi"("error in (no error)"=w21, "Channel in"=w22) -> ("error out"=→"error out":errorcluster, "Channel out"=w20:refnum<class "Channel.lvclass">)  [unwired: 8 in]
  n122 = flat-sequence {
    tunnel: w20 -> [_]
    frame #0 {
      w282 = ""
      w286 = FALSE
      w288 = FALSE ("Acquiring")
      w294 = 0.0
      w295 = 1024.0
      w289 = u16 0 ("Cubes done")
      n123 = local write "Acquiring"(FALSE ("Acquiring")) -> ()
      n124 = local write "Serial number"(u16 0 ("Serial number")) -> ()
      n125 = local write "CCD status"("" ("CCD status")) -> ()
      n126 = local write "Last image"("" ("Last image")) -> ()
      n127 = local write "cycles done"(w289) -> ()
      n128 = local write "CCD ON/OFF"(FALSE ("CCD ON/OFF")) -> ()
      n129 = local write "Temperature status"("" ("Temperature status")) -> ()
      n130 = local write "frames done"(u16 0 ("Frames done")) -> ()
      n131 = local write "seqs done"(w289) -> ()
      n132 = local write "Error Message"("") -> ()
      n133 = local write "Numeric"(0 ("Numeric")) -> ()
      n134 = local write "Acquiring 2"(FALSE ("Acquiring 2")) -> ()
      n135 = local write "exptime (s)"(0.0 ("Frame exptime (s)")) -> ()
      n136 = local write "Temperature (ºC)"(i16 0 ("Current temperature (ºC)")) -> ()
      n137 = property on="Intensity Graph" class="IntGraph (strict)"("ZScale.Maximum"=30000.0, "ZScale.Minimum"=0.0) -> ()  [unwired: 2 in, 2 out]
      n138 = property on="Intensity Graph" class="IntGraph (strict)"("XScale.Maximum"=w295, "XScale.Minimum"=w294, "YScale.Maximum"=w295, "YScale.Minimum"=w294) -> ()  [unwired: 2 in, 2 out]
      n139 = local write "counts level"(15.0) -> ()
      n140 = local write "contrast"(1.0) -> ()
      n141 = local write "Header CCD Config"(T3 {"EM_GAIN"=0, "FRAME_TRANSFER"=FALSE, "SHUTTER_OPENING_TIME"=0, "SHUTTER_CLOSING_TIME"=0, "VBIN"=0, "INITIAL_LINE"=0, "INITIAL_COLUMN"=0, "FINAL_LINE"=0, "FINAL_COLUMN"=0, "HBIN"=0, "AD_CHANNEL"=0, "EM_MODE"=1, "PREAMP"=0, "SHUTTER_TTL"=0, "SHUTTER_MODE"=2, "ACQUISITION_MODE"=3, "TRIGGER_MODE"=0, "VERTICAL_CLOCK_VOLTAGE"=0, "VERTICAL_SHIFT_SPEED"=3, "READ_MODE"=4, "Last update"=timestamp(0 s since 1904-01-01), "READOUT_RATE"=""} ("Header CCD Config")) -> ()
      n142 = local write "Wait expose cmd"(w288) -> ()
      n143 = local write "video mode"(w288) -> ()
      n144 = local write "S4GUI"(w286) -> ()
      n145 = local write "S4ICS"(w286) -> ()
      n146 = local write "TCS"(w286) -> ()
      n147 = local write "Weather Station"(w286) -> ()
      n148 = local write "Focuser"(w286) -> ()
      n149 = local write "S4GUI"(w282) -> ()
      n150 = local write "S4ICS"(w282) -> ()
      n151 = local write "TCS"(w282) -> ()
      n152 = local write "Focuser"(w282) -> ()
      n153 = local write "Weather station"(w282) -> ()
      n154 = local write "ACS status"(w282) -> ()
    }
  }
